vi "写入通信句柄.vi"(8 "error in (no error)":errorcluster, 10 "通信句柄":variant, 11 "串口通信类 in":refnum<class "串口通信类.lvclass">) -> (0 "error out":errorcluster, 3 "串口通信类 out":refnum<class "串口通信类.lvclass">)   [LabVIEW 2015, in "串口通信类.lvclass"]
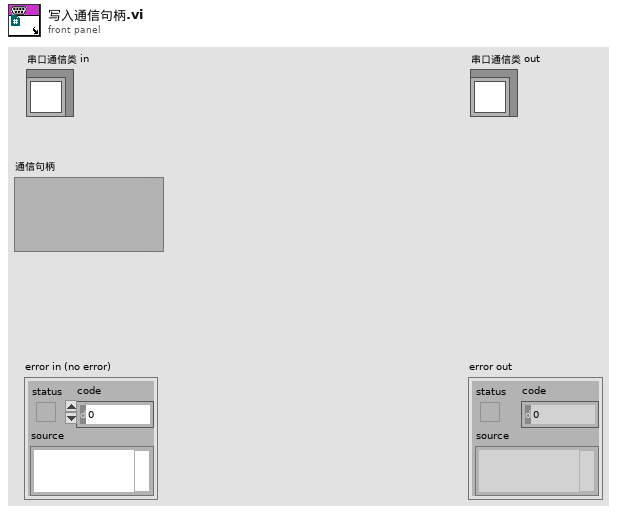
[diagram p1: front panel]
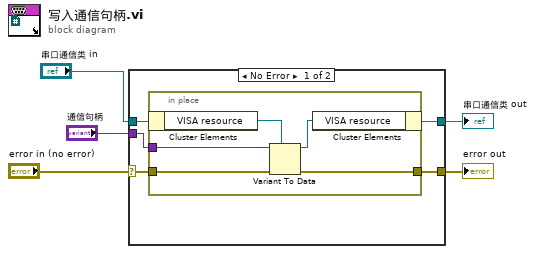
[diagram p0: block diagram]
diagram:
  n1 = case shown="No Error" "error in (no error)" {
    selector: "error in (no error)" -> [w8 w17]
    tunnel: "通信句柄" -> [w10 _]
    tunnel: "串口通信类 in" -> [w9 w16]
    tunnel: [w7 w17] -> w2
    tunnel: [w6 w16] -> w1
    frame No Error {
      n2 = in-place "In Place Element Structure" {
        in-place-border: w10 -> [w15]
        in-place-border: w8 -> [w12]
        in-place-border: [w11] -> w7
        n3 = in-place-cluster #1(w9) -> ("VISA resource"=w14:refnum<visa-resource-name>)
        n4 = Variant To Data(error in=w12, type=w14, Variant=w15) -> (data=w13:refnum<visa-resource-name>, error out=w11:errorcluster)
        n5 = in-place-cluster #1("VISA resource"=w13) -> (w6:refnum<class "串口通信类.lvclass">)
      }
    }
    frame Error {
    }
  }
  "error out" <- w2
  "串口通信类 out" <- w1
